vi "Execute.vi"(8 "error in (no error)":errorcluster, 11 "Buy Stock Order in":refnum<class "Buy Stock Order.lvclass">) -> (0 "error out":errorcluster, 3 "Order Out":refnum<class "Order.lvclass">)   [LabVIEW 2019, in "Buy Stock Order.lvclass"]
doc: "Execute the Buy action (Concrete Command) on the Stock Trade (Reciever)"
uses:
  Buy Stock Order.lvclass
  C:/Users/Tiba/Desktop/Command Pattern 2014/Command Pattern 2014/Order/Order.lvclass
  Order/Order.lvclass
  Buy Stock Order.lvclass/Buy Stock Order.ctl
  Stock Trader/Stock Trader.lvclass
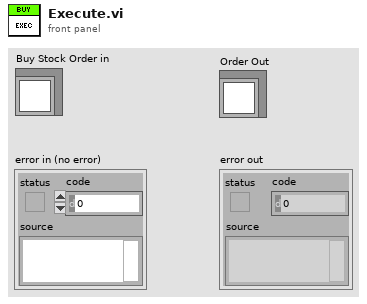
[diagram p1: front panel]
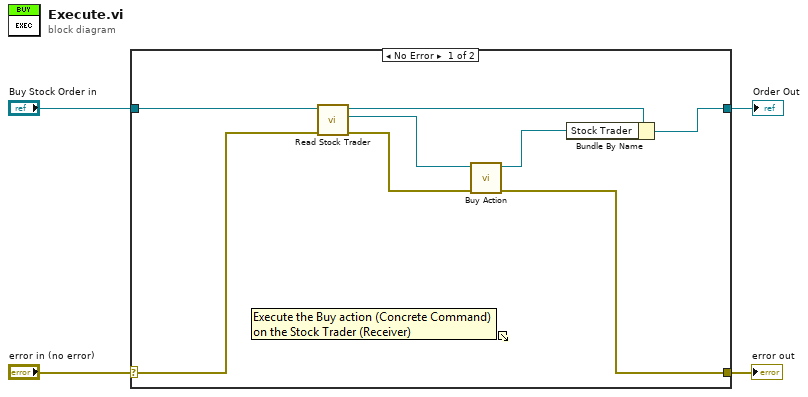
[diagram p0: block diagram]
diagram:
  n1 = case shown="No Error" "error in (no error)" {
    selector: "error in (no error)" -> [w10 w14]
    tunnel: [w8 w14] -> w3
    tunnel: [w5 w13] -> w1
    tunnel: "Buy Stock Order in" -> [w12 w13]
    frame No Error {
      n2 = call-dynamic "Read Stock Trader.vi"("error in (no error)"=w10, "Order in"=w12) -> ("error out"=w9:errorcluster, "Stock Trader"=w11:refnum<class "Stock Trader.lvclass">, "Order out"=w6:refnum<class "Buy Stock Order.lvclass">)  [unwired: 7 in]
      n3 = call "Buy Action.vi"("error in (no error)"=w9, "Stock Trader In"=w11) -> ("error out"=w8:errorcluster, "Stock Trader Out"=w7:refnum<class "Stock Trader.lvclass">)  [unwired: 8 in]
      n4 = Bundle By Name(cluster=w6, "Stock Trader"=w7) -> (w5:refnum<class "Buy Stock Order.lvclass">)
    }
    frame Error {
    }
  }
  "error out" <- w3
  "Order Out" <- w1
